vi "NicmosPostFirstTelemetry.vi"(7 "Synchronization":T1, 9 "error in (no error)":errorcluster) -> (6 "error out":errorcluster)   [LabVIEW 2009]
uses:
  Controls/NicmosSynchronization.ctl
  Controls/NICMOS.COMMAND.ctl
  Controls/NICMOS.COMMANDBASIC.ctl
  Controls/NICMOS.READOUT.ctl
  Controls/NICMOS.FILTERCOMMAND.ctl
  Controls/NICMOS.FILTER.ctl
  Controls/NICMOS.STATE.ctl
  Controls/NICMOS.DATA.ctl
  Controls/NICMOS.RAW.ctl
  Controls/NICMOS.TEMPERATURE.ctl
  Controls/NICMOS.MASKBANKS.ctl
  <vilib>/Utility/config.llb/NI_LVConfig.lvlib
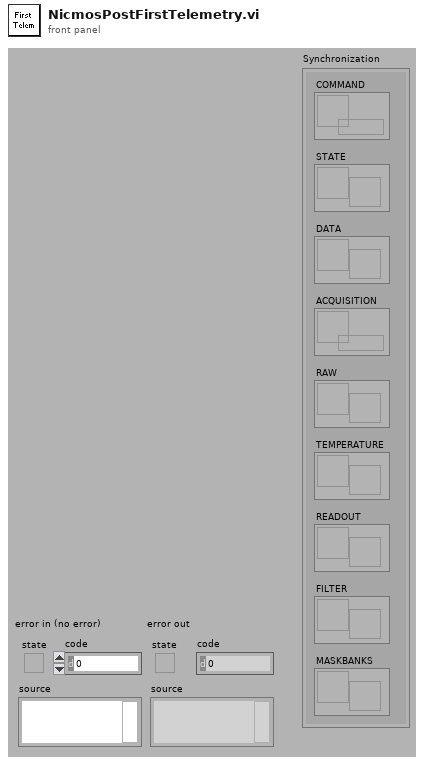
[diagram p1: front panel]
types:
  T1 = typedef "NicmosSynchronization.ctl" = cluster{"COMMAND":refnum<queue>, "STATE":refnum<notifier>, "DATA":refnum<notifier>, "ACQUISITION":refnum<queue>, "RAW":refnum<notifier>, "TEMPERATURE":refnum<notifier>, "READOUT":refnum<notifier>, "FILTER":refnum<notifier>, "MASKBANKS":refnum<notifier>}
  T2 = typedef "NICMOS.MASKBANKS.ctl" = cluster{"MaskList":cluster{"X":i32, "Y":i32, "NX":i32, "NY":i32}[], "Reform X":i32, "Reform Y":i32}[]
  T3 = typedef "NICMOS.FILTER.ctl" = string
  T4 = typedef "NI_LVConfig.lvlib/Config Data RefNum.ctl" = refnum<k1>
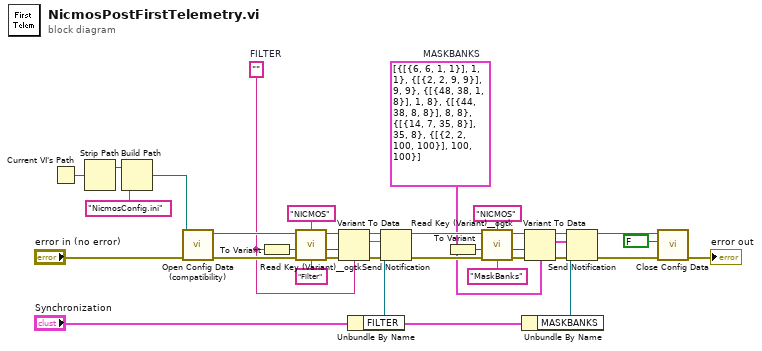
[diagram p0: block diagram]
diagram:
  w2 = T2 [{"MaskList"=[{"X"=6, "Y"=6, "NX"=1, "NY"=1}], "Reform X"=1, "Reform Y"=1}, {"MaskList"=[{"X"=2, "Y"=2, "NX"=9, "NY"=9}], "Reform X"=9, "Reform Y"=9}, {"MaskList"=[{"X"=48, "Y"=38, "NX"=1, "NY"=8}], "Reform X"=1, "Reform Y"=8}, {"MaskList"=[{"X"=44, "Y"=38, "NX"=8, "NY"=8}], "Reform X"=8, "Reform Y"=8}, {"MaskList"=[{"X"=14, "Y"=7, "NX"=35, "NY"=8}], "Reform X"=35, "Reform Y"=8}, {"MaskList"=[{"X"=2, "Y"=2, "NX"=100, "NY"=100}], "Reform X"=100, "Reform Y"=100}]  # MASKBANKS
  w7 = T3 ""  # FILTER
  n1 = Current VI's Path() -> (path=w32:path)
  n2 = Strip Path(path=w32) -> (stripped path=w25:path)  [unwired: 1 out]
  n3 = Build Path(base path=w25, name or relative path="NicmosConfig.ini" ("nom ou chemin relatif")) -> (appended path=w30:path)
  n4 = call <vilib>:"Open Config Data (compatibility).vi"("error in (no error)"="error in (no error)", "configuration file path"=w30) -> ("error out"=w29:errorcluster, "refnum"=w28:T4)  [unwired: 7 in, 1 out]
  n5 = To Variant(anything=w7) -> (Variant=w12:variant)
  n6 = call <userlib>:"Read Key (Variant)__ogtk.vi"("section"="NICMOS", "error in (no error)"=w29, "type"=w12, "key (optional)"="Filter" ("key"), "refnum"=w28) -> ("error out"=w10:errorcluster, "key-value"=w8:variant, "refnum out"=w22:T4)  [unwired: 3 in, 1 out]
  n7 = Variant To Data(error in=w10, Variant=w8, type=w7) -> (error out=w9:errorcluster, data=w6:T3)
  n8 = Unbundle By Name("Synchronization") -> ("FILTER"=w26:refnum<notifier>)
  n9 = Send Notification(notification=w6, notifier=w26, error in (no error)=w9) -> (error out=w23:errorcluster)  [unwired: 1 out]
  n10 = To Variant(anything=w2) -> (Variant=w11:variant)
  n11 = call <userlib>:"Read Key (Variant)__ogtk.vi"("section"="NICMOS", "error in (no error)"=w23, "type"=w11, "key (optional)"="MaskBanks" ("key"), "refnum"=w22) -> ("error out"=w4:errorcluster, "key-value"=w5:variant, "refnum out"=w19:T4)  [unwired: 3 in, 1 out]
  n12 = Unbundle By Name("Synchronization") -> ("MASKBANKS"=w24:refnum<notifier>)
  n13 = Variant To Data(error in=w4, Variant=w5, type=w2) -> (error out=w3:errorcluster, data=w1:T2)
  n14 = Send Notification(notification=w1, notifier=w24, error in (no error)=w3) -> (error out=w20:errorcluster)  [unwired: 1 out]
  n15 = call <vilib>:"Close Config Data.vi"("error in (no error)"=w20, "write file if changed (T)"=FALSE ("write configuration file? (T)"), "refnum"=w19) -> ("error out"=→"error out":errorcluster)  [unwired: 7 in, 1 out]
